vi "Test.vi"() -> ()   [LabVIEW 2015, in "Blinker.lvclass"]
uses:
  Blinker.lvclass
  Blinker.lvclass/Blinker.ctl
panel:
  out "State":bool
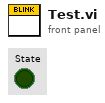
[diagram p1: front panel]
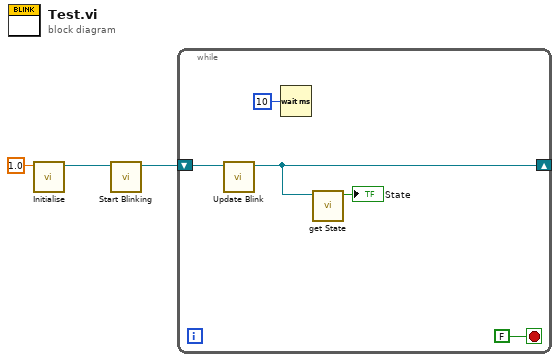
[diagram p0: block diagram]
diagram:
  n1 = call "Initialise.vi"("Blink Period [s]"=1.0 ("Blink Period")) -> ("Blink out"=w2:refnum<class "Blinker.lvclass">)  [unwired: 10 in]
  n2 = call "Start Blinking.vi"("Blinker in"=w2) -> ("Blinker out"=w1:refnum<class "Blinker.lvclass">)  [unwired: 10 in]
  n3 = while {
    shift-right: [w7] -> _
    shift-left: w1 -> [w8]
    stop <- FALSE stop-if-true
    n4 = call "Update Blink.vi"("Blinker in"=w8) -> ("Blinker out"=w7:refnum<class "Blinker.lvclass">)  [unwired: 10 in]
    n5 = Wait (ms)(milliseconds to wait=u32 10) -> ()  [unwired: 1 out]
    n6 = call "get State.vi"("Blinker in"=w7) -> ("Blink State"=→"State":bool)  [unwired: 10 in]
  }
